vi "PROGRA 16.vi"() -> ()   [LabVIEW 2011]
panel:
  in  "stop":bool
  in  "Suma":bool
  out "Menor":dbl
  out "Mayor":dbl
  out "Promedio":dbl
  out "Suma":dbl
  out "Array":dbl[](array[numeric])
  in  "Generar":bool
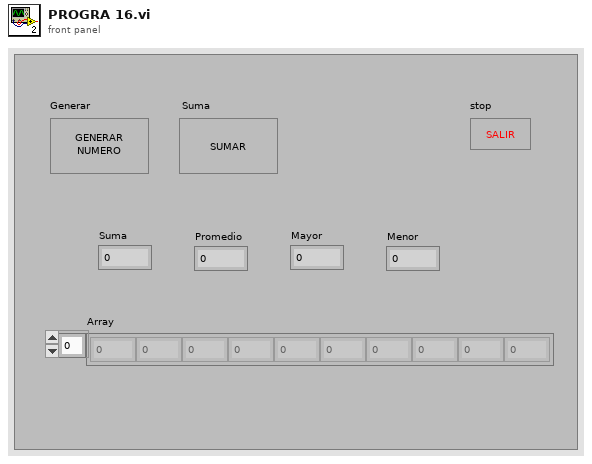
[diagram p1: front panel]
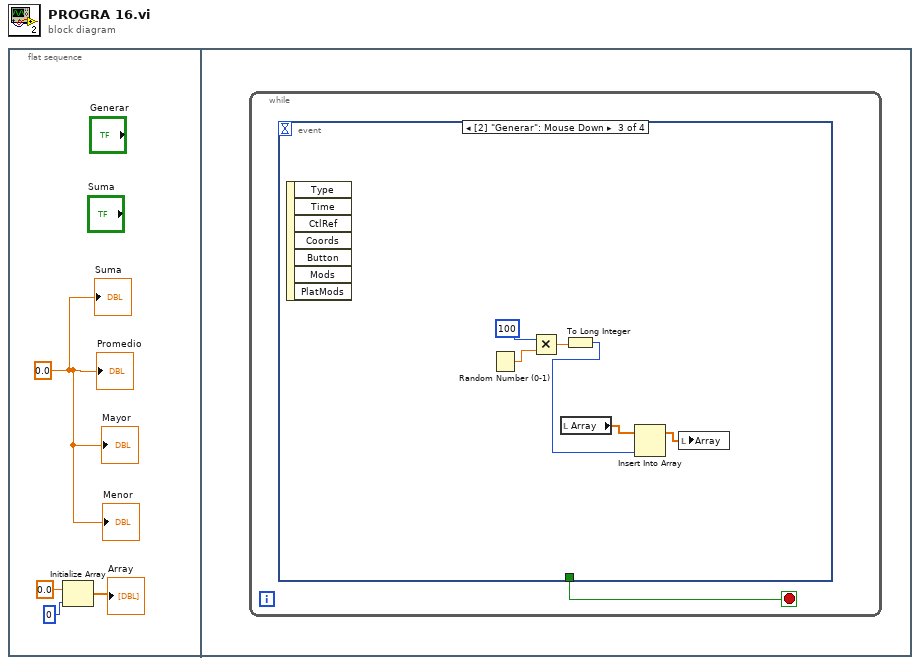
[diagram p0: block diagram]
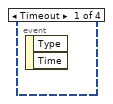
[diagram p2: hidden frame]
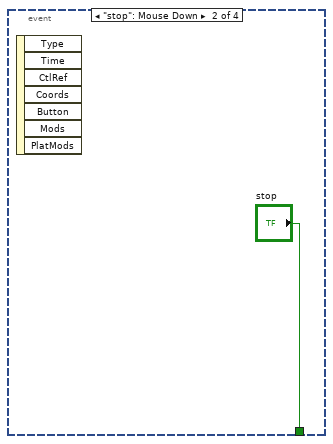
[diagram p3: hidden frame]
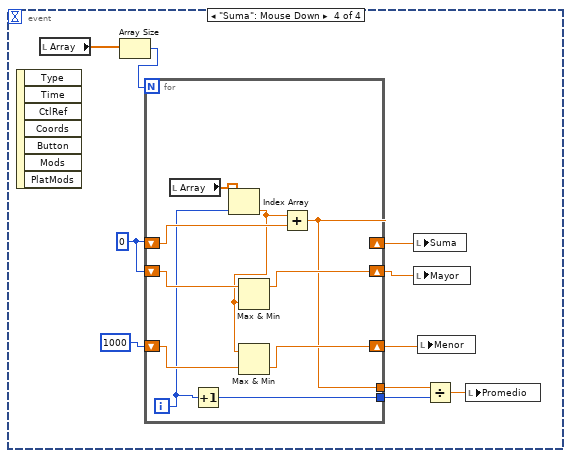
[diagram p4: hidden frame]
diagram:
  n1 = flat-sequence {
    frame #0 {
      w4 = 0.0 ("Promedio")
      n2 = Initialize Array(0.0 ("element"), 0 ("dimension size")) -> (→"Array":dbl[])
      "Suma" <- w4
      "Promedio" <- w4
      "Mayor" <- w4
      "Menor" <- w4
    }
    frame #1 {
      n3 = while {
        stop <- w5 stop-if-true
        n4 = event shown="[2] \"Generar\": Mouse Down" {
          selector: _ -> [_ _ _ _]
          dyn-events: _ -> [_ _ _ _]
          timeout: _ -> [_ _ _ _]
          tunnel: [_ "stop" _ _] -> w5
          event Timeout {
            n5 = event-data() -> ()  [unwired: 1 in, 2 out]
          }
          event "stop": Mouse Down {
            n6 = event-data() -> ()  [unwired: 1 in, 7 out]
          }
          event "Generar": Mouse Down {
            n7 = event-data() -> ()  [unwired: 1 in, 7 out]
            n8 = Random Number (0-1)() -> (number: 0 to 1=w12:dbl)
            n9 = Multiply(x=100, y=w12) -> (x*y=w10:dbl)
            n10 = local read "Array"() -> (w9:dbl[])
            n11 = To Long Integer(number=w10) -> (32bit integer=w8:i32)
            n12 = Insert Into Array "Insert Into Array"(array=w9, new element=w8) -> (w7:dbl[])  [unwired: 1 in]
            n13 = local write "Array"(w7) -> ()
          }
          event "Suma": Mouse Down {
            w19 = 0 ("dimension size")
            n14 = event-data() -> ()  [unwired: 1 in, 7 out]
            n15 = local read "Array"() -> (w21:dbl[])
            n16 = Array Size(array=w21) -> (size(s)=w22:i32)
            n17 = for {
              N: w22 -> [_]
              shift-right: [w23] -> w20
              shift-left: w19 -> [w31]
              shift-right: [w29] -> w18
              shift-left: w19 -> [w30]
              shift-right: [w27] -> w16
              shift-left: 1000 ("dimension size") -> [w28]
              tunnel: [w25] -> w15
              tunnel: [w23] -> w14
              i -> [w26]
              n18 = local read "Array"() -> (w32:dbl[])
              n19 = Increment(x=w26) -> (x+1=w25:i32)
              n20 = Index Array(array=w32, index=w26) -> (element=w24:dbl)
              n21 = Max & Min(x=w30, y=w24) -> (max(x,y)=w29:dbl)  [unwired: 1 out]
              n22 = Max & Min(x=w24, y=w28) -> (min(x,y)=w27:dbl)  [unwired: 1 out]
              n23 = Add(x=w24, y=w31) -> (x+y=w23:dbl)
            }
            n24 = local write "Suma"(w20) -> ()
            n25 = local write "Mayor"(w18) -> ()
            n26 = local write "Menor"(w16) -> ()
            n27 = Divide(x=w14, y=w15) -> (x/y=w13:dbl)
            n28 = local write "Promedio"(w13) -> ()
          }
        }
      }
    }
  }
